vi "Get Control Ref by Name.vi"(8 "error in (no error)":errorcluster, 10 "Name":string, 11 "VI Ref":refnum<vi>) -> (0 "error out":errorcluster, 1 "Owning Pane":refnum<vi>, 2 "Ctl Ref":refnum<vi>, 3 "VI Ref out":refnum<vi>)   [LabVIEW 2020, in "MacroAssert.lvlib"]
doc: "Outputs a reference for the control with <B>Name</B> from the VI identified by <B>VI Ref</B>."
uses:
  MacroAssert.lvlib
  Custom Errors/Custom Errors.lvlib
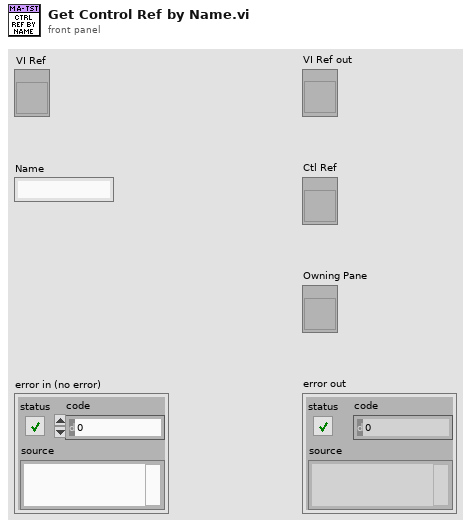
[diagram p1: front panel]
types:
  T1 = typedef "MacroAssert.lvlib/Control Map Control Data.ctl" = cluster{"Owner Labels":string[], "Owner Classes":string[], "Ctl Ref":refnum<vi>, "Owning Pane":refnum<vi>}
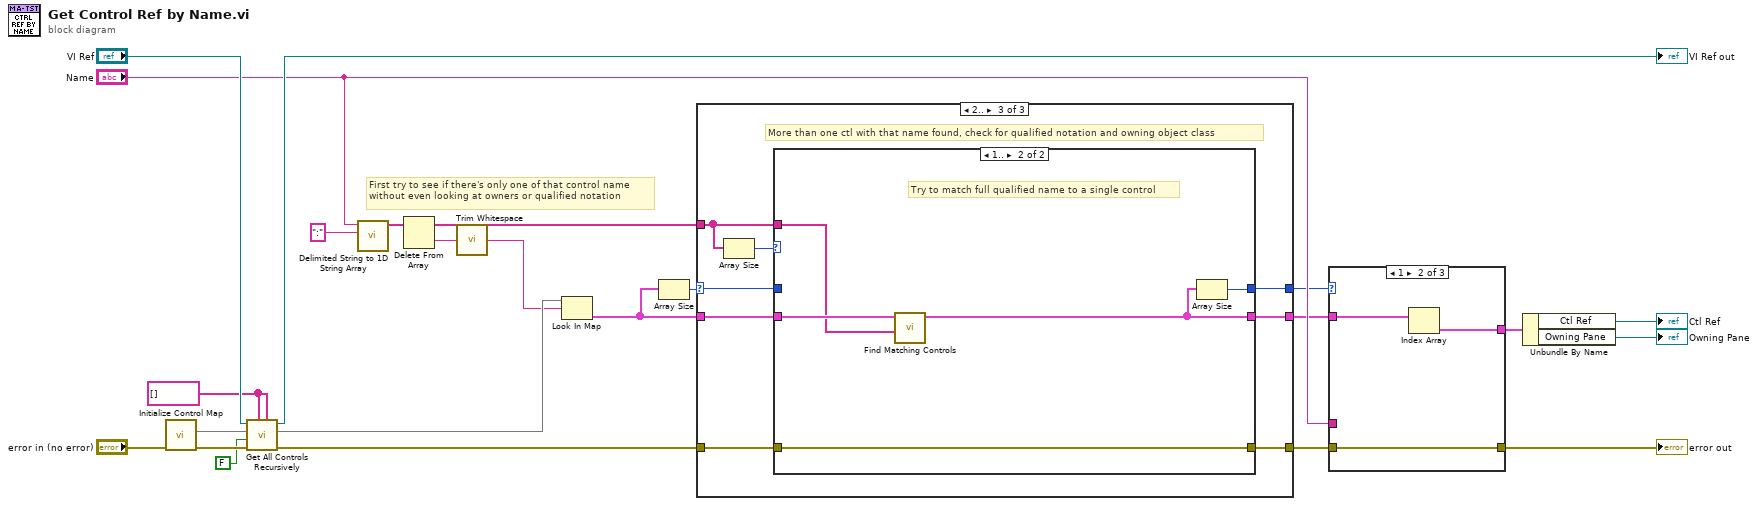
[diagram p0: block diagram]
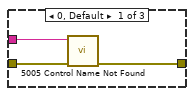
[diagram p2: hidden frame]
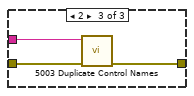
[diagram p3: hidden frame]
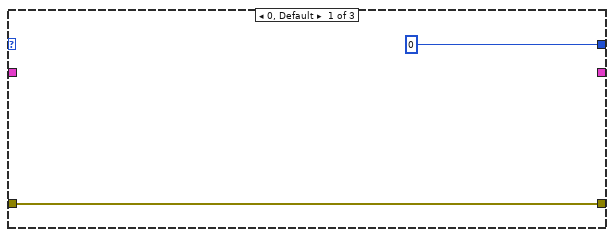
[diagram p4: hidden frame]
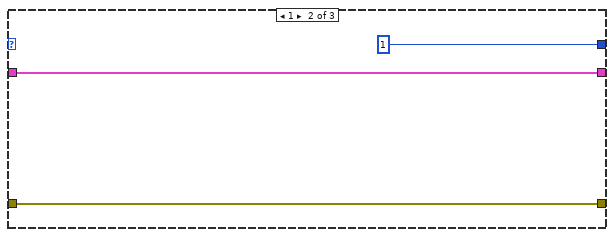
[diagram p5: hidden frame]
diagram:
  w9 = string[] [] ("Owner Classes")
  # "First try to see if there's only one of that control name without even looking at owners or qualified notation"
  n1 = call "Initialize Control Map.vi"("error in (no error)"="error in (no error)") -> ("error out"=w12:errorcluster, "Control Map"=w11:map{string, T1[]})  [unwired: 9 in]
  n2 = call "Get All Controls Recursively.vi"("Owner Labels"=w9, "Owner Classes"=w9, "error in (no error)"=w12, "Subpanel?"=FALSE, "Control Map"=w11, "VI Ref"="VI Ref") -> ("error out"=w19:errorcluster, "Control Map out"=w6:map{string, T1[]}, "VI Ref out"=→"VI Ref out":refnum<vi>)  [unwired: 3 in]
  n3 = call <vilib>:"Delimited String to 1D String Array.vi"("delimiter"=":", "delimited string"="Name") -> ("string array"=w18:string[])  [unwired: 9 in]
  n4 = Delete From Array(array=w18) -> (deleted portion=w8:string, array with subset deleted=w1:string[])  [unwired: 2 in]
  n5 = call <vilib>:"Trim Whitespace.vi"("string"=w8) -> ("trimmed string"=w2:string)  [unwired: 1 in]
  n6 = Look In Map(map=w6, key=w2) -> (value=w7:T1[])  [unwired: 1 in, 1 out]
  n7 = Array Size(array=w7) -> (size(s)=w21:i32)
  n8 = case shown="2.." w21 {
    selector: w21 -> [_ _ w31]
    tunnel: w7 -> [_ w27 w37]
    tunnel: [_ w27 w33] -> w14
    tunnel: [w26 w29 w35] -> w15
    tunnel: w19 -> [w26 w29 w36]
    tunnel: w1 -> [_ _ w34]
    tunnel: [0 1 w32] -> w16
    frame 0, Default {
    }
    frame 1 {
    }
    frame 2.. {
      # "More than one ctl with that name found, check for qualified notation and owning object class"
      n9 = Array Size(array=w34) -> (size(s)=w30:i32)
      n10 = case shown="1.." w30 {
        tunnel: w37 -> [_ w42]
        tunnel: w36 -> [w39 w44]
        tunnel: [w39 w44] -> w35
        tunnel: w34 -> [_ w41]
        tunnel: [_ w40] -> w33
        tunnel: [w38 w43] -> w32
        tunnel: w31 -> [w38 _]
        frame 0, Default {
          # "No qualified notation specified to be able to look at ctl owners, just report that duplicates were found"
        }
        frame 1.. {
          # "Try to match full qualified name to a single control"
          n11 = call "Find Matching Controls.vi"("Qualified Name Array"=w41, "Ctl Data"=w42) -> ("Ctl Data out"=w40:T1[])  [unwired: 9 in]
          n12 = Array Size(array=w40) -> (size(s)=w43:i32)
        }
      }
    }
  }
  n13 = case shown="1" w16 {
    tunnel: w14 -> [_ w50 _]
    tunnel: [_ w49 _] -> w5
    tunnel: w15 -> [w47 w48 w53]
    tunnel: "Name" -> [w46 _ w51]
    tunnel: [w45 w48 w52] -> w13
    frame 0, Default {
      n14 = call "5005 Control Name Not Found.vi"("error in (no error)"=w47, "Control Name"=w46) -> ("error out"=w45:errorcluster)  [unwired: 9 in]
    }
    frame 1 {
      n15 = Index Array(array=w50) -> (element=w49:T1)  [unwired: 1 in]
    }
    frame 2 {
      n16 = call "5003 Duplicate Control Names.vi"("error in (no error)"=w53, "Control Name"=w51) -> ("error out"=w52:errorcluster)  [unwired: 9 in]
    }
  }
  "error out" <- w13
  n17 = Unbundle By Name(w5) -> ("Ctl Ref"=→"Ctl Ref":refnum<vi>, "Owning Pane"=→"Owning Pane":refnum<vi>)
